vi "4461 Sim - Noise.vi"(8 "error in (no error)":errorcluster, 9 "AO []":waveform(dbl)[](array[waveform]), 11 "Lockin":refnum<class "Instrument.Lockin.lvclass">) -> (0 "error out":errorcluster, 2 "\"AI\" []":waveform(dbl)[](array[waveform]), 3 "Lockin out":refnum<class "Instrument.Lockin.lvclass">)   [LabVIEW 2016, in "LockinDAQ.lvclass"]
uses:
  LockinDAQ.lvclass
  <vilib>/measure/NI_MABase.lvlib
  <vilib>/Analysis/NI_AALPro.lvlib
  <vilib>/Analysis/2dsp.llb/Inverse Real FFT.vi
  <vilib>/Analysis/NI_AALBase.lvlib
  <vilib>/Analysis/3filter.llb/Butterworth Filter (DBL).vi
  <vilib>/Analysis/2dsp.llb/Real FFT.vi
  Instrument.Lockin/Instrument.Lockin.lvclass
  C:/Program Files (x86)/National Instruments/LabVIEW 2016/user.lib/LevyLab/Levylab Instruments/SMOs/Instrument/Instrument.lvclass
  C:/Program Files (x86)/National Instruments/LabVIEW 2016/user.lib/LevyLab/Levylab Instruments/SMOs/LevyLab/LevyLab.lvclass
  C:/Program Files (x86)/National Instruments/LabVIEW 2016/vi.lib/JKI/JKI SMO/SMO/SMO.lvclass
panel:
  in  "Noise Cluster":T1={"1/f vs. Uniform "=1.0, "DC Drift Fraction"=0.0, "DC Drift Freq"=0.19999999999999996, "DC Offset"=0.0, "60Hz Amplitude"=0.005, "Gauss/Unif %"=0.5, "Sig Amp"=1.0, "Noise Amp"=0.005}
  out "Signal Graph":waveform(dbl)[](graph)
  out "Noisy Signal Graph":waveform(dbl)[](graph)
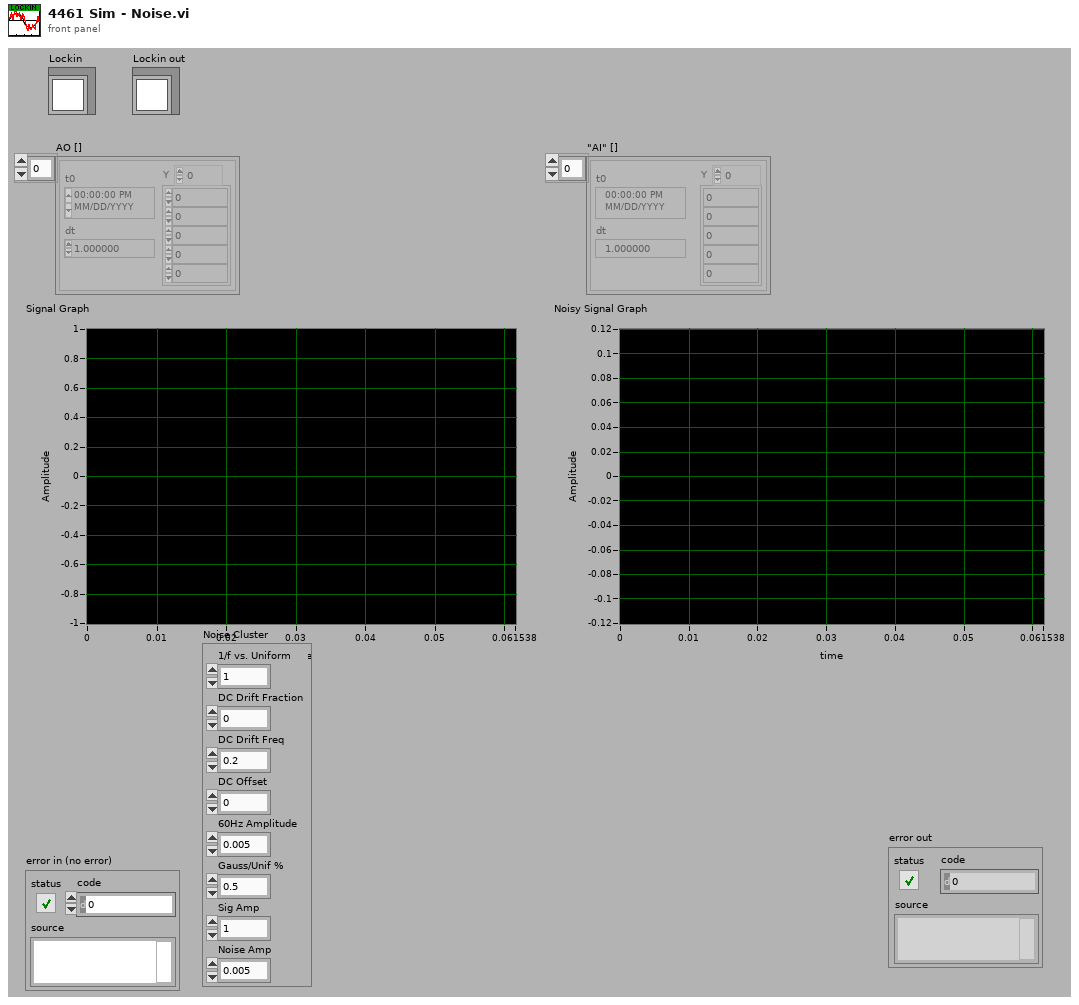
[diagram p1: front panel]
types:
  T1 = cluster{"1/f vs. Uniform ":dbl, "DC Drift Fraction":dbl, "DC Drift Freq":dbl, "DC Offset":dbl, "60Hz Amplitude":dbl, "Gauss/Unif %":dbl, "Sig Amp":dbl, "Noise Amp":dbl}
  T2 = enum32{"Lowpass", "Highpass", "Bandpass", "Bandstop"}
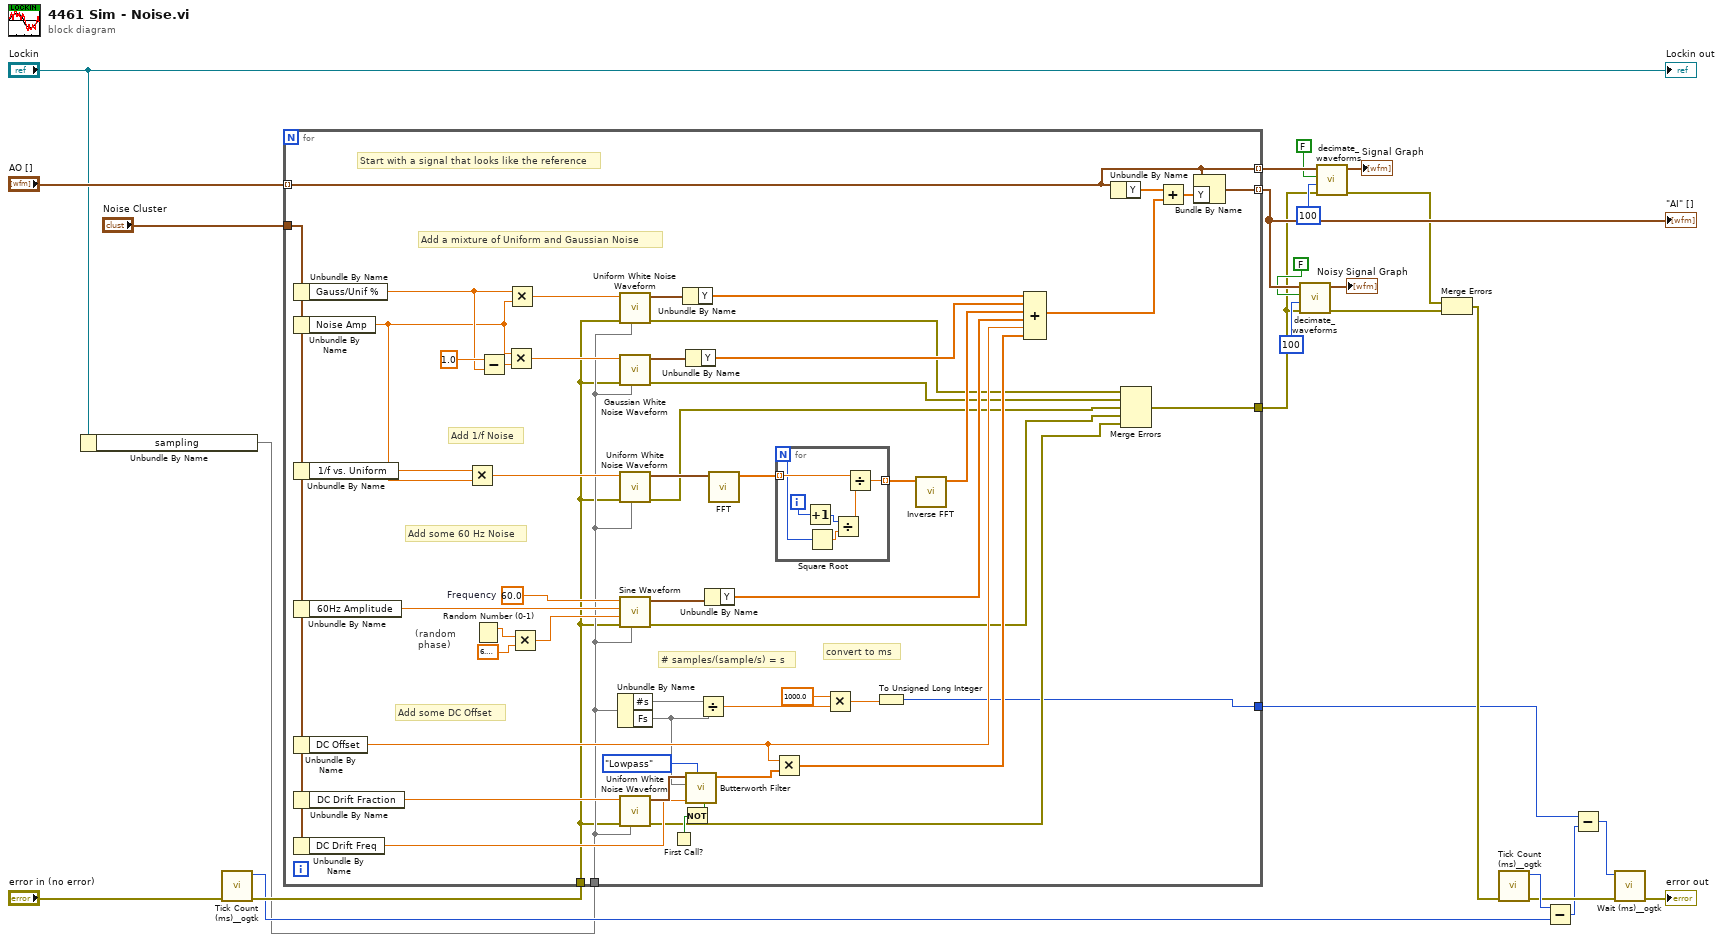
[diagram p0: block diagram]
diagram:
  n1 = Unbundle By Name("Lockin") -> ("sampling"=w1)
  n2 = call <userlib>:"Tick Count (ms)__ogtk.vi"("error in (no error)"="error in (no error)") -> ("error out"=w13:errorcluster, "millisecond timer value"=w8:u32)  [unwired: 9 in]
  n3 = for {
    tunnel: "Noise Cluster" -> [w44]
    tunnel: w1 -> [w37]
    tunnel: "AO []" -> [w40] mode=indexing
    tunnel: [w47] -> w24 mode=indexing
    tunnel: [w27] -> w5
    tunnel: [w40] -> w18 mode=indexing
    tunnel: w13 -> [w36]
    tunnel: [w30] -> w16
    w38 = 60.0  # Frequency
    # "convert to ms"
    # "# samples/(sample/s) = s"
    # "Start with a signal that looks like the reference"
    # "Add 1/f Noise"
    # "(random\n phase)"
    # "Add some DC Offset"
    # "Add some 60 Hz Noise"
    # "Add a mixture of Uniform and Gaussian Noise"
    n4 = Unbundle By Name(w44) -> ("Gauss/Unif %"=w56:dbl)
    n5 = Unbundle By Name(w44) -> ("Noise Amp"=w54:dbl)
    n6 = Unbundle By Name(w44) -> ("1/f vs. Uniform"=w55:dbl)
    n7 = Unbundle By Name(w44) -> ("60Hz Amplitude"=w53:dbl)
    n8 = Unbundle By Name(w44) -> ("DC Offset"=w52:dbl)
    n9 = Unbundle By Name(w44) -> ("DC Drift Fraction"=w50:dbl)
    n10 = Unbundle By Name(w44) -> ("DC Drift Freq"=w51:dbl)
    n11 = Multiply(x=w55, y=w54) -> (x*y=w64:dbl)
    n12 = Random Number (0-1)() -> (number: 0 to 1=w72:dbl)
    n13 = Subtract(x=1.0, y=w56) -> (x-y=w75:dbl)
    n14 = Multiply(x=w54, y=w75) -> (x*y=w43:dbl)
    n15 = Multiply(x=w56, y=w54) -> (x*y=w42:dbl)
    n16 = Multiply(x=w72, y=6.283185307179586) -> (x*y=w41:dbl)
    n17 = Unbundle By Name(w37) -> ("#s"=w46, "Fs"=w45)
    n18 = call <vilib>:"Uniform White Noise Waveform.vi"("sampling info"=w37, "error in (no error)"=w36, "amplitude"=w42) -> ("error out"=w35:errorcluster, "signal out"=w76:waveform(dbl))  [unwired: 7 in]
    n19 = call <vilib>:"Gaussian White Noise Waveform.vi"("sampling info"=w37, "error in (no error)"=w36, "standard deviation"=w43) -> ("error out"=w34:errorcluster, "signal out"=w77:waveform(dbl))  [unwired: 7 in]
    n20 = call <vilib>:"Uniform White Noise Waveform.vi"("sampling info"=w37, "error in (no error)"=w36, "amplitude"=w64) -> ("error out"=w33:errorcluster, "signal out"=w63:waveform(dbl))  [unwired: 7 in]
    n21 = call <vilib>:"Sine Waveform.vi"("sampling info"=w37, "error in (no error)"=w36, "phase"=w41, "amplitude"=w53, "frequency"=w38) -> ("error out"=w32:errorcluster, "signal out"=w71:waveform(dbl))  [unwired: 5 in]
    n22 = call <vilib>:"Uniform White Noise Waveform.vi"("sampling info"=w37, "error in (no error)"=w36, "amplitude"=w50) -> ("error out"=w31:errorcluster, "signal out"=w70:waveform(dbl))  [unwired: 7 in]
    n23 = First Call?() -> (First Call?: T/F=w57:bool)
    n24 = Not(x=w57) -> (.not. x?=w68:bool)
    n25 = Unbundle By Name(w76) -> ("Y"=w66:dbl[])
    n26 = Unbundle By Name(w77) -> ("Y"=w58:dbl[])
    n27 = call-poly <vilib>:"Butterworth Filter.vi"("init/cont (init:F)"=w68, "filter type"=T2."Lowpass", "low cutoff freq: fl"=w51, "sampling freq: fs"=w45, "X"=w70) -> ("Filtered X"=w67:dbl[])  [unwired: 3 in, 1 out]
    n28 = Divide(x=w46, y=w45) -> (x/y=w26:dbl)
    n29 = Unbundle By Name(w71) -> ("Y"=w62:dbl[])
    n30 = call-poly <vilib>:"FFT.vi"("X"=w63) -> ("FFT {X}"=w39:cdb[])  [unwired: 9 in, 1 out]
    n31 = Multiply(x=w52, y=w67) -> (x*y=w60:dbl[])
    n32 = for {
      N -> [w81]
      tunnel: [w84] -> w65 mode=indexing
      tunnel: w39 -> [w83] mode=indexing
      i -> [w82]
      n33 = Increment(x=w82) -> (x+1=w79:i32)
      n34 = Square Root(x=w81) -> (sqrt(x)=w80:dbl)
      n35 = Divide(x=w79, y=w80) -> (x/y=w78:dbl)
      n36 = Divide(x=w83, y=w78) -> (x/y=w84:cdb)
    }
    n37 = Multiply(x=1000.0, y=w26) -> (x*y=w28:dbl)
    n38 = To Unsigned Long Integer(number=w28) -> (unsigned 32bit integer=w27:u32)
    n39 = call-poly <vilib>:"Inverse FFT.vi"("FFT {X}"=w65) -> ("X"=w61:dbl[])  [unwired: 9 in, 1 out]
    n40 = Compound Arithmetic op=ADD(w66, w58, w61, w62, w52, w60) -> (w59:dbl[])
    n41 = Unbundle By Name(w40) -> ("Y"=w49:dbl[])
    n42 = Merge Errors(w35, w34, w33, w32, w31) -> (w30:errorcluster)
    n43 = Add(x=w49, y=w59) -> (x+y=w48:dbl[])
    n44 = Bundle By Name(cluster=w40, "Y"=w48) -> (w47:waveform(dbl))
  }
  "\"AI\" []" <- w24
  n45 = call "decimate_waveforms.vi"("Input Signal"=w24, "averaging"=FALSE, "decimating factor"=100, "error in (no error)"=w16) -> ("Decimated Waveforms"=→"Noisy Signal Graph":waveform(dbl)[], "error out"=w15:errorcluster)  [unwired: 5 in]
  n46 = call "decimate_waveforms.vi"("Input Signal"=w18, "averaging"=FALSE, "decimating factor"=100, "error in (no error)"=w16) -> ("Decimated Waveforms"=→"Signal Graph":waveform(dbl)[], "error out"=w11:errorcluster)  [unwired: 5 in]
  n47 = Merge Errors(w11, w15) -> (w10:errorcluster)
  n48 = call <userlib>:"Tick Count (ms)__ogtk.vi"("error in (no error)"=w10) -> ("error out"=w7:errorcluster, "millisecond timer value"=w9:u32)  [unwired: 9 in]
  n49 = Subtract(x=w9, y=w8) -> (x-y=w3:u32)
  n50 = Subtract(x=w5, y=w3) -> (x-y=w4:u32)
  n51 = call <userlib>:"Wait (ms)__ogtk.vi"("error in (no error)"=w7, "milliseconds to wait"=w4) -> ("error out"=→"error out":errorcluster)  [unwired: 8 in, 1 out]
  "Lockin out" <- "Lockin"
